vi "Pass.vi"(7 "Caller":string, 8 "error in (no error)":errorcluster, 10 "Assertion":string) -> (0 "error out":errorcluster)   [LabVIEW 2017, in "Caraya Adapter.lvclass"]
uses:
  Caraya Adapter.lvclass
  <vilib>/addons/_JKI Toolkits/Caraya/classes/Assert/Assert.lvclass
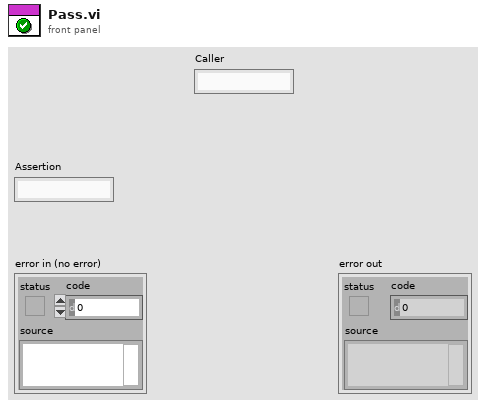
[diagram p1: front panel]
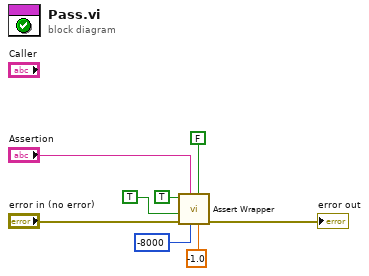
[diagram p0: block diagram]
diagram:
  n1 = call <vilib>:"Assert Wrapper.vi"("Execution time (s)"=-1.0, "Assert Only? (F)"=FALSE, "error code (1)"=-8000, "Label"="Assertion", "error in (no error)"="error in (no error)", "Register with caller test (F)"=TRUE, "Assert?"=TRUE) -> ("error out"=→"error out":errorcluster)  [unwired: 1 in, 3 out]
